vi "Generate Image.vi"(8 "error in (no error)":errorcluster, 11 "Camera Simulator in":refnum<class "Camera Simulator.lvclass">) -> (0 "error out":errorcluster, 3 "Camera Simulator out":refnum<class "Camera Simulator.lvclass">)   [LabVIEW 2020, in "Camera Simulator.lvlib" / "Camera Simulator.lvclass"]
uses:
  Camera Simulator.lvclass
  Camera Simulator.lvclass/Camera Simulator.ctl
  <vilib>/vision/NI_Vision_Development_Module.lvlib
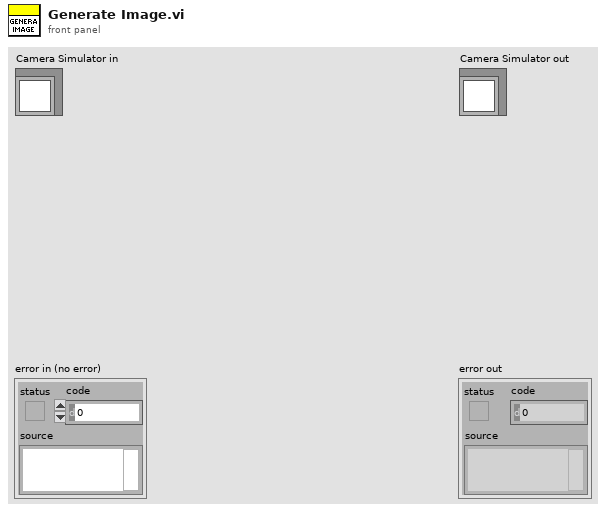
[diagram p1: front panel]
types:
  T1 = typedef "IMAQ Image.ctl" = refnum<image>
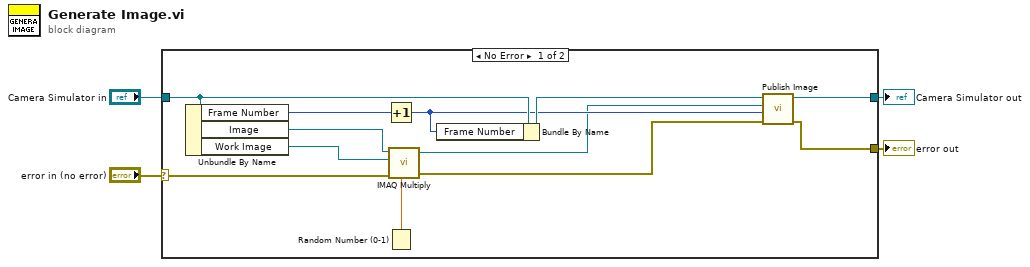
[diagram p0: block diagram]
diagram:
  n1 = case shown="No Error" "error in (no error)" {
    selector: "error in (no error)" -> [w15 w18]
    tunnel: [w13 w18] -> w3
    tunnel: [w14 w17] -> w1
    tunnel: "Camera Simulator in" -> [w16 w17]
    frame No Error {
      n2 = Unbundle By Name(w16) -> ("Frame Number"=w11:u32, "Image"=w8:T1, "Work Image"=w7:T1)
      n3 = Increment(x=w11) -> (x+1=w10:u32)
      n4 = Random Number (0-1)() -> (number: 0 to 1=w5:dbl)
      n5 = call "IMAQ Multiply"("Image Src A"=w8, "Constant"=w5, "Image Dst"=w7, "error in (no error)"=w15) -> ("Image Dst Out"=w6:T1, "error out"=w9:errorcluster)  [unwired: 3 in]
      n6 = Bundle By Name(cluster=w16, "Frame Number"=w10) -> (w12:refnum<class "Camera Simulator.lvclass">)
      n7 = call-dynamic "Publish Image.vi"("error in (no error)"=w9, "Buffer Number"=w10, "Image"=w6, "Camera in"=w12) -> ("error out"=w13:errorcluster, "Camera out"=w14:refnum<class "Camera Simulator.lvclass">)  [unwired: 6 in]
    }
    frame Error {
    }
  }
  "error out" <- w3
  "Camera Simulator out" <- w1
